vi "MFC Polling Loop.vi"(11 "MFC Actor.lvlib:MFC.lvclass":refnum<class "MFC.lvclass">) -> ()   [LabVIEW 2018, in "MFC Actor.lvlib" / "MFC.lvclass"]
uses:
  MFC.lvclass
  C:/Program Files/National Instruments/LabVIEW 2018/vi.lib/MGI/Panel Manager/Panel Actor/Panel Actor/Panel Actor.lvclass
  <vilib>/ActorFramework/Message Enqueuer/Message Enqueuer.lvclass/Message Enqueuer.ctl
  <vilib>/ActorFramework/Message Enqueuer/Enqueue.vi
  MFC Messages/Read Flow Msg/Read Flow Msg.lvclass
  C:/Program Files/National Instruments/LabVIEW 2018/vi.lib/ActorFramework/Message/Message.lvclass
  <vilib>/ActorFramework/Message Priority Queue/Priority Enqueue.vi
  <vilib>/MGI/Panel Manager/Panel Actor/Panel Actor/Panel Actor.lvclass
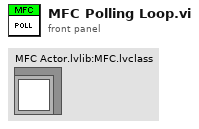
[diagram p1: front panel]
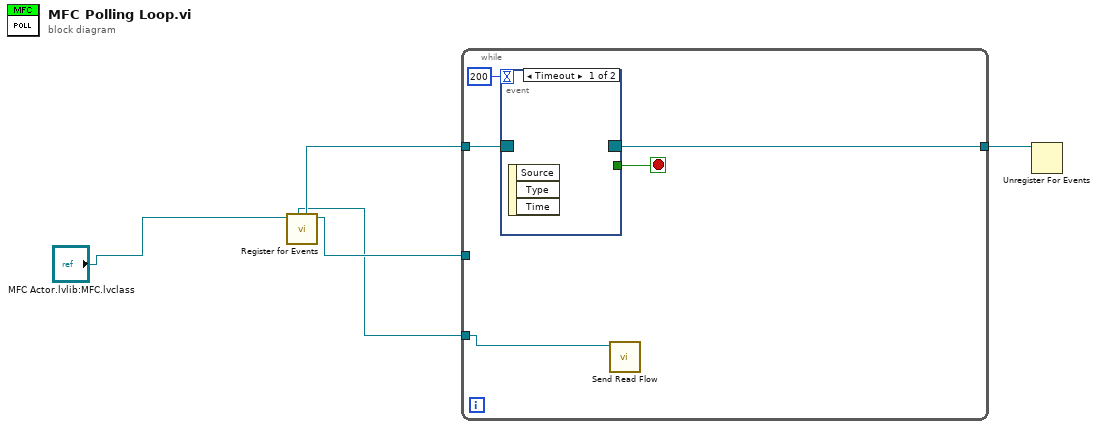
[diagram p0: block diagram]
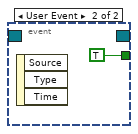
[diagram p2: hidden frame]
diagram:
  n1 = call <vilib>:"Register for Events.vi"("Panel Actor in"="MFC Actor.lvlib:MFC.lvclass") -> ("Panel Actor out"=w4:refnum<class "MFC.lvclass">, "Pnl Actor"=w3:refnum<event-registration>, "Self Enqueuer"=w1:refnum<class "Message Enqueuer.lvclass">)  [unwired: 7 in, 1 out]
  n2 = while {
    tunnel: w3 -> [w10]
    tunnel: [w9] -> w5
    tunnel: w1 -> [w7]
    tunnel: w4 -> [_]
    stop <- w8 stop-if-true
    n3 = event shown="[0] Timeout" {
      selector: w10 -> [_ _]
      dyn-events: [_ _] -> w9
      timeout: 200 -> [_ _]
      tunnel: [_ TRUE] -> w8
      event Timeout {
        n4 = event-data() -> ()  [unwired: 1 in, 3 out]
      }
      event User Event {
        n5 = event-data() -> ()  [unwired: 1 in, 3 out]
      }
    }
    n6 = call "Send Read Flow.vi"("Message Enqueuer"=w7) -> ()  [unwired: 9 in, 2 out]
  }
  n7 = Unregister For Events(event registration refnum=w5) -> ()  [unwired: 1 in, 1 out]
